vi "zmq tcp data latency - data reply.vi"() -> ()   [LabVIEW 2019]
uses:
  <vilib>/addons/zeromq/socket_type.ctl
  <vilib>/addons/zeromq/zmq_context.lvclass
  <vilib>/addons/zeromq/zmq_socket.lvclass
  <vilib>/addons/zeromq/zeromq.lvlib
panel:
  in  "endpoint":string="tcp://*:5555"
  out "Numeric":i32
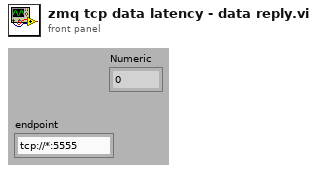
[diagram p1: front panel]
types:
  T1 = typedef "zeromq.lvlib/socket_type.ctl" = enum8{"ZMQ_PAIR", "ZMQ_PUB", "ZMQ_SUB", "ZMQ_REQ", "ZMQ_REP", "ZMQ_DEALER", "ZMQ_ROUTER", "ZMQ_PULL", "ZMQ_PUSH", "ZMQ_XPUB", "ZMQ_XSUB"}
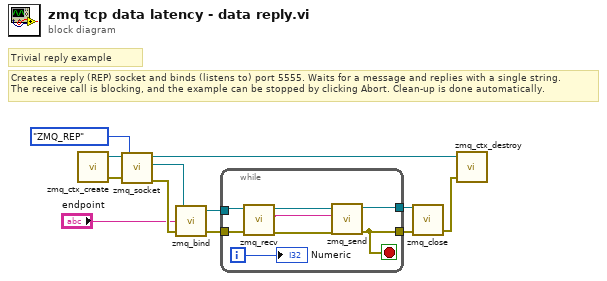
[diagram p0: block diagram]
diagram:
  # "Creates a reply (REP) socket and binds (listens to) port 5555. Waits for a message and replies with a single string.\nThe receive call is blocking, and the example can be stopped by clicking Abort. Clean-up is done automatically."
  # "Trivial reply example"
  n1 = call <vilib>:"zmq_ctx_create.vi"() -> ("error out"=w10:errorcluster, "context out"=w9:refnum<class "zmq_context.lvclass">)  [unwired: 4 in]
  n2 = call <vilib>:"zmq_socket.vi"("error in"=w10, "socket type"=socket_type."ZMQ_REP", "context in"=w9) -> ("error out"=w12:errorcluster, "socket out"=w11:refnum<class "zmq_socket.lvclass">, "context out"=w1:refnum<class "zmq_context.lvclass">)  [unwired: 2 in]
  n3 = call <vilib>:"zmq_bind.vi"("error in"=w12, "endpoint"="endpoint", "socket in"=w11) -> ("error out"=w5:errorcluster, "socket out"=w6:refnum<class "zmq_socket.lvclass">)  [unwired: 1 in]
  n4 = while {
    tunnel: w6 -> [w19]
    tunnel: w5 -> [w20]
    tunnel: [w16] -> w4
    tunnel: [w15] -> w3
    i -> [w13]
    stop <- w16 stop-if-true
    n5 = call <vilib>:"zmq_recv.vi"("error in"=w20, "socket in"=w19) -> ("error out"=w18:errorcluster, "data"=w14:string, "socket out"=w17:refnum<class "zmq_socket.lvclass">)  [unwired: 3 in, 2 out]
    n6 = call <vilib>:"zmq_send.vi"("error in"=w18, "data"=w14, "socket in"=w17) -> ("error out"=w16:errorcluster, "socket out"=w15:refnum<class "zmq_socket.lvclass">)  [unwired: 4 in]
    "Numeric" <- w13
  }
  n7 = call <vilib>:"zmq_close.vi"("error in"=w4, "socket"=w3) -> ("error out"=w2:errorcluster)  [unwired: 3 in]
  n8 = call <vilib>:"zmq_ctx_destroy.vi"("error in"=w2, "context in"=w1) -> ()  [unwired: 3 in, 1 out]
